vi "Read.vi"(8 "error in (no error)":errorcluster, 11 "DMM in":refnum<class "DMM.lvclass">) -> (0 "error out":errorcluster, 1 "String":string, 2 "Measurement":dbl format="%.5f", 3 "DMM out":refnum<class "DMM.lvclass">)   [LabVIEW 2012, in "DMM.lvclass"]
uses:
  DMM.lvclass
  DMM.lvclass/DMM.ctl
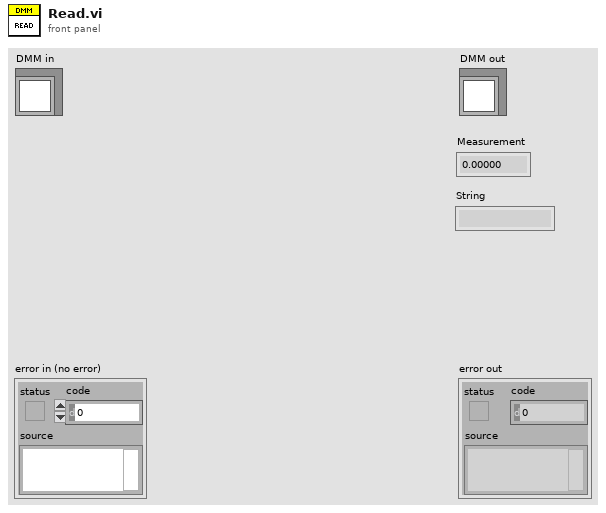
[diagram p1: front panel]
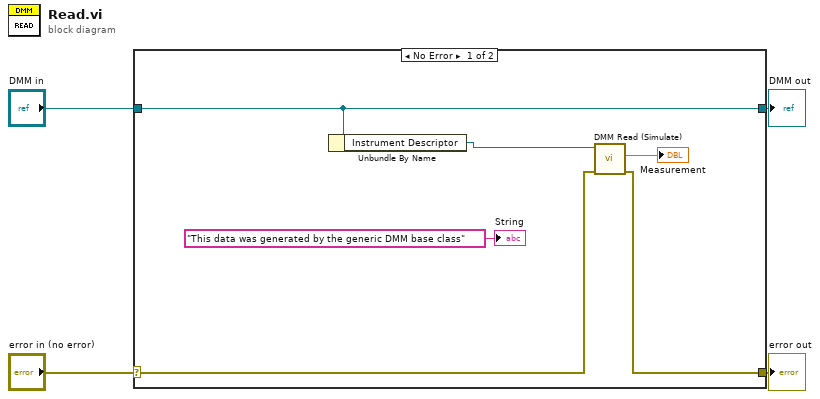
[diagram p0: block diagram]
diagram:
  n1 = case shown="No Error" "error in (no error)" {
    selector: "error in (no error)" -> [w7 w12]
    tunnel: [w6 w12] -> w3
    tunnel: [w9 w11] -> w1
    tunnel: "DMM in" -> [w9 w11]
    frame No Error {
      n2 = Unbundle By Name(w9) -> ("Instrument Descriptor"=w8:refnum<visa-resource-name>)
      n3 = call "DMM Read (Simulate).vi"("error in (no error)"=w7, "Instrument Refnum in"=w8) -> ("error out"=w6:errorcluster, "Measurement"=→"Measurement":dbl)  [unwired: 7 in, 1 out]
      "String" <- "This data was generated by the generic DMM base class" ("String")
    }
    frame Error {
    }
  }
  "error out" <- w3
  "DMM out" <- w1
